vi "Wizard Status Update.vi"(2 "Cluster in":cluster{u32, string}, 3 "String":string) -> (0 "Cluster out":cluster{u32, string})   [LabVIEW 2014]
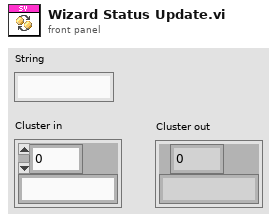
[diagram p1: front panel]
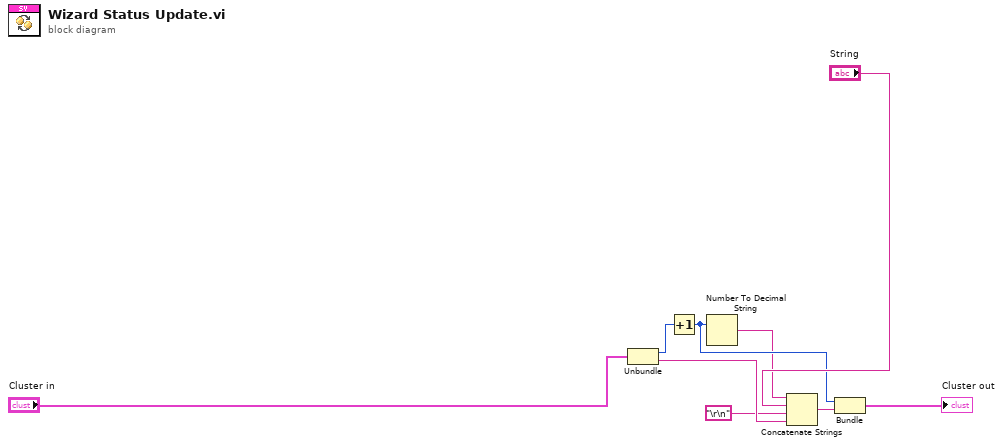
[diagram p0: block diagram]
diagram:
  n1 = Unbundle("Cluster in") -> (w5:u32, w3:string)
  n2 = Increment(x=w5) -> (x+1=w6:u32)
  n3 = Number To Decimal String(number=w6) -> (decimal integer string=w2:string)  [unwired: 1 in]
  n4 = Concatenate Strings(w2, "String", "\r\n", w3) -> (w4:string)
  n5 = Bundle(w6, w4) -> (→"Cluster out":cluster{u32, string})  [unwired: 1 in]
